vi "Motor_ControllerIdle.vi"(6 "Reinitialize":bool, 8 "error in (no error)":errorcluster, 11 "Motor Control in":refnum<class "MotorControl.lvclass">) -> (0 "error out":errorcluster, 2 "VoltageCommand":dbl[](array[numeric]) format="%.2f", 3 "Motor Control out":refnum<class "MotorControl.lvclass">)   [LabVIEW 2015, in "MotorControl.lvclass"]
uses:
  MotorControl.lvclass
  MotorControl.lvclass/MotorControl.ctl
  <vilib>/addons/control/pid/pid.llb/PID Output Rate Limiter (DBL Array).vi
  <vilib>/addons/control/pid/NI_PID_pid.lvlib
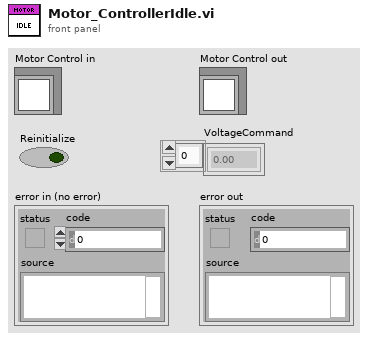
[diagram p1: front panel]
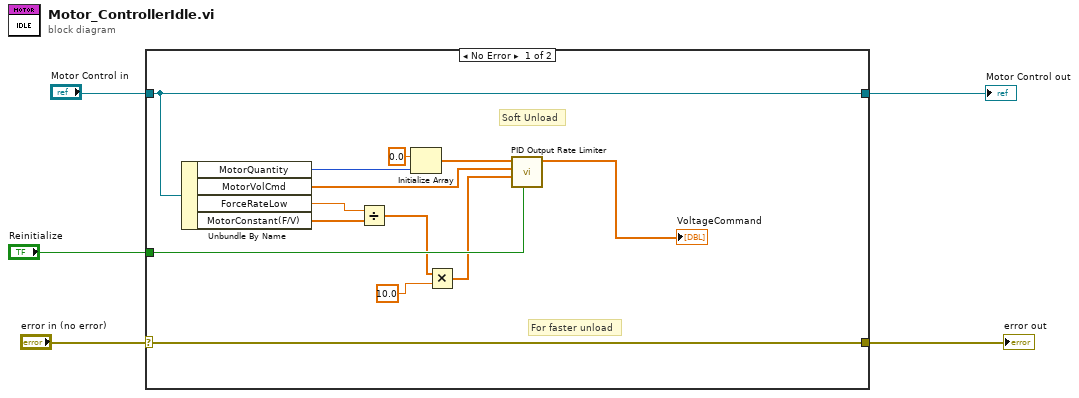
[diagram p0: block diagram]
diagram:
  n1 = case shown="No Error" "error in (no error)" {
    selector: "error in (no error)" -> [w10 w19]
    tunnel: [w9 w20] -> w5
    tunnel: [w10 w19] -> w4
    tunnel: "Motor Control in" -> [w9 w20]
    tunnel: "Reinitialize" -> [w17 _]
    frame No Error {
      # "For faster unload"
      # "Soft Unload"
      n2 = Unbundle By Name(w9) -> ("MotorQuantity"=w14:i32, "MotorVolCmd"=w15:dbl[], "ForceRateLow"=w13:dbl, "MotorConstant(F/V)"=w12:dbl[])
      n3 = Divide(x=w13, y=w12) -> (x/y=w8:dbl[])
      n4 = Initialize Array(0.0 ("element"), w14) -> (w16:dbl[])
      n5 = Multiply(x=w8, y=10.0 ("element")) -> (x*y=w7:dbl[])
      n6 = call-poly <vilib>:"PID Output Rate Limiter.vi"("reinitialize? (F)"=w17, "output rate (EGU/min)"=w7, "initial output"=w15, "input (controller output)"=w16) -> ("output"=→"VoltageCommand":dbl[])  [unwired: 4 in, 1 out]
    }
    frame Error {
    }
  }
  "Motor Control out" <- w5
  "error out" <- w4
